vi "Query SR830 sensitivity.vi"(8 "error in (no error)":errorcluster caption="错误输入（无错误）", 11 "VISA resource name":refnum<visa-resource-name>) -> (0 "错误输出":errorcluster, 2 "sensitivity":i32, 3 "VISA resource name out":refnum<visa-resource-name>)   [LabVIEW 2019, in "User lib.lvlib"]
uses:
  User lib.lvlib
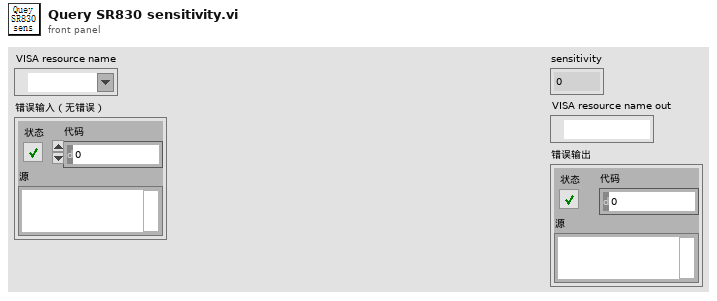
[diagram p1: front panel]
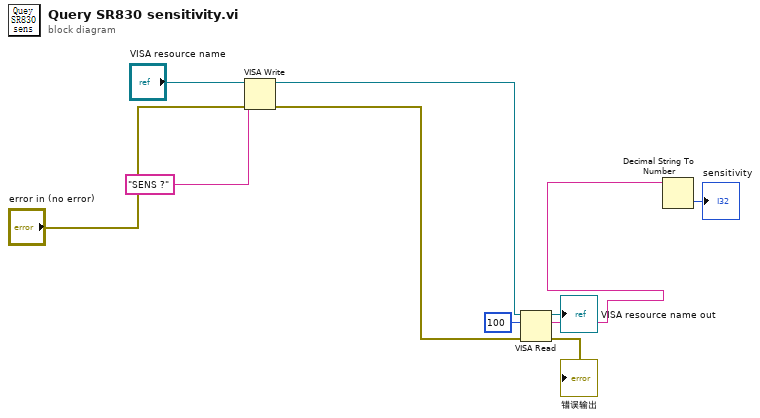
[diagram p0: block diagram]
diagram:
  n1 = VISA Write(VISA resource name="VISA resource name", write buffer="SENS ?" ("写入缓冲区"), error in (no error)="error in (no error)") -> (VISA resource name out=w7:refnum<visa-resource-name>, error out=w6:errorcluster)  [unwired: 1 out]
  n2 = VISA Read(VISA resource name=w7, byte count=u32 100 ("字节总数"), error in (no error)=w6) -> (VISA resource name out=→"VISA resource name out":refnum<visa-resource-name>, read buffer=w3:string, error out=→"错误输出":errorcluster)  [unwired: 1 out]
  n3 = Decimal String To Number(string=w3) -> (number=→"sensitivity":i32)  [unwired: 2 in, 1 out]
